vi "Helmholtz2D_Solve Lin Sys_Apply Corner.vi"(6 "Boundary Condition":cluster{"type":T2, "Value":dbl[]}[](array[cluster]) {"type" items=["Dirichlet", "Neumann"]}, 7 "Domain":T3={"x"={"start x"=0.0, "end x"=1.0, "# of x-points"=11}, "y"={"start y"=0.0, "end y"=1.0, "# of y-points"=11}}, 10 "D":T1, 11 "C'":T1) -> (0 "D' End Y":T1, 1 "D' Start Y":T1, 2 "C' End Y":T1, 3 "C' Start Y":T1)   [LabVIEW 2017, in "NI_PDE.lvlib"]
uses:
  <vilib>/gmath/NI_PDE.lvlib
  <vilib>/Analysis/Matrix/Datatypes/RealMatrix.ctl
  <vilib>/gmath/pde.llb/Common/PDE_BC Type.ctl
  <vilib>/Analysis/7linalg.llb/Create Special Real Matrix.vi
  <vilib>/Analysis/NI_AALPro.lvlib
  <vilib>/Analysis/Matrix/NI_Matrix.lvlib
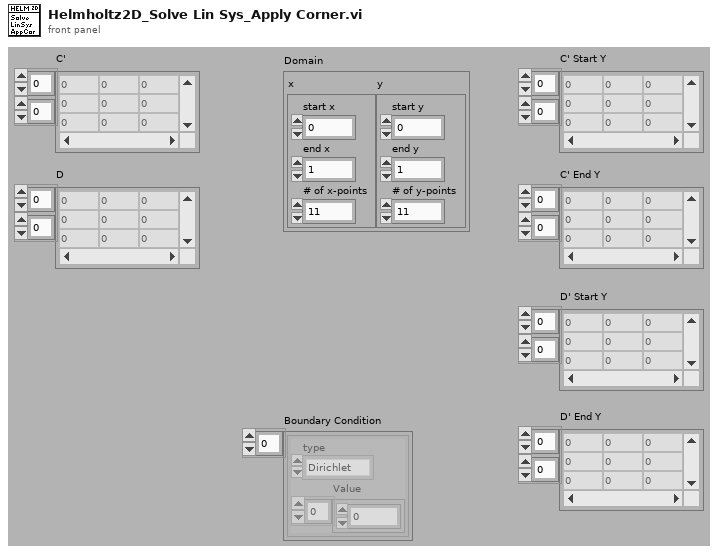
[diagram p1: front panel]
types:
  T1 = typedef "NI_Matrix.lvlib/RealMatrix.ctl" = dbl[][]
  T2 = typedef "NI_PDE.lvlib/PDE_BC Type.ctl" = i32
  T3 = cluster{"x":cluster{"start x":dbl, "end x":dbl, "# of x-points":i32}, "y":cluster{"start y":dbl, "end y":dbl, "# of y-points":i32}}
  T4 = enum32{"Identity", "Diagonal", "Toepliz", "Vandermonde", "Companion"}
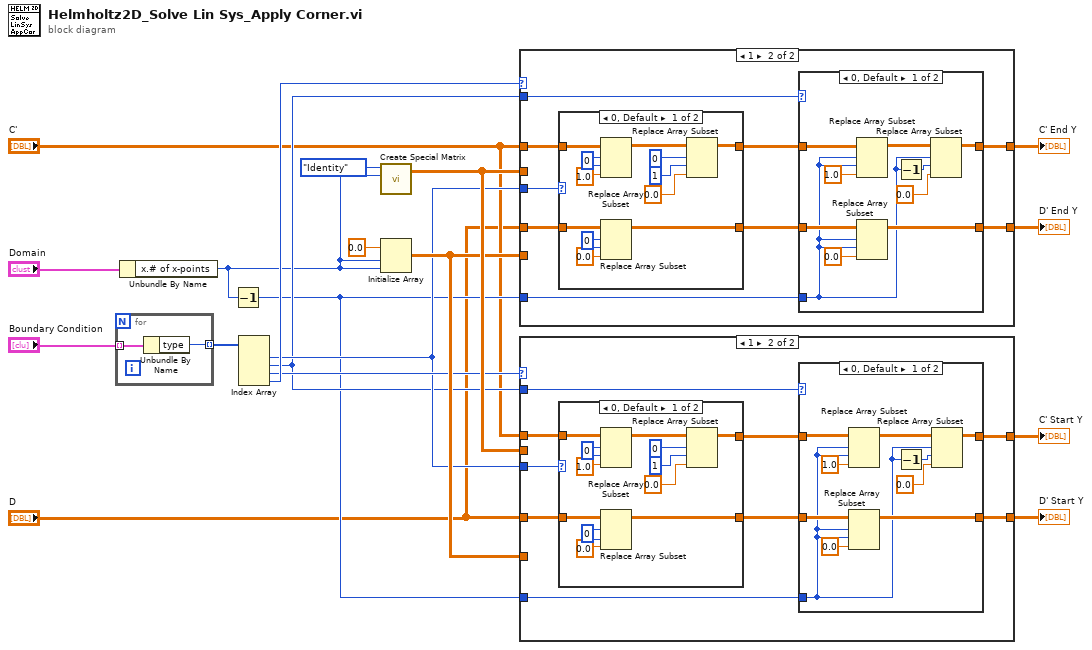
[diagram p0: block diagram]
diagram:
  n1 = for {
    tunnel: "Boundary Condition" -> [w21] mode=indexing
    tunnel: [w20] -> w9 mode=indexing
    n2 = Unbundle By Name(w21) -> ("type"=w20:T2)
  }
  n3 = Unbundle By Name("Domain") -> ("x.# of x-points"=w1:i32)
  n4 = Decrement(x=w1) -> (x-1=w4:i32)
  n5 = Index Array(array=w9) -> (element #1=w6:T2, element #2=w5:T2, element #3=w7:T2, element #4=w8:T2)  [unwired: 4 in]
  n6 = call-poly <vilib>:"Create Special Matrix.vi"("matrix type"=T4."Identity", "matrix size"=w1) -> ("Special Matrix"=w15:T1)  [unwired: 2 in, 2 out]
  n7 = Initialize Array(0.0 ("element"), w1, w1) -> (w14:dbl[][])
  n8 = case shown="1" w8 {
    tunnel: w15 -> [w23 _]
    tunnel: [w23 w27] -> w13
    tunnel: "C'" -> [_ w31]
    tunnel: w6 -> [_ w32]
    tunnel: "D" -> [_ w30]
    tunnel: [w22 w25] -> w12
    tunnel: w14 -> [w22 _]
    tunnel: w5 -> [_ w29]
    tunnel: w4 -> [_ w24]
    frame 0, Default {
    }
    frame 1 {
      n9 = case shown="0, Default" w32 {
        tunnel: w31 -> [w49 w58]
        tunnel: [w46 w58] -> w28
        tunnel: [w54 w57] -> w26
        tunnel: w30 -> [w55 w57]
        frame 0, Default {
          w48 = 0 ("index (row)")
          w45 = 0 ("index (row)")
          n10 = Replace Array Subset(array=w49, new element=1.0 ("new element/subarray"), index (row)=w48, index (col)=w48) -> (w47:T1)
          n11 = Replace Array Subset(array=w55, new element=0.0 ("new element/subarray"), index (row)=w45, index (col)=w45) -> (w54:T1)
          n12 = Replace Array Subset(array=w47, new element=0.0 ("new element/subarray"), index (row)=0, index (col)=1 ("index (row)")) -> (w46:T1)
        }
        frame 1 {
        }
      }
      n13 = case shown="0, Default" w29 {
        tunnel: w28 -> [w37 w44]
        tunnel: [w35 w44] -> w27
        tunnel: [w40 w43] -> w25
        tunnel: w26 -> [w41 w43]
        tunnel: w24 -> [w33 _]
        frame 0, Default {
          n14 = Replace Array Subset(array=w37, new element=1.0 ("new element/subarray"), index (row)=w33, index (col)=w33) -> (w36:T1)
          n15 = Replace Array Subset(array=w41, new element=0.0 ("new element/subarray"), index (row)=w33, index (col)=w33) -> (w40:T1)
          n16 = Decrement(x=w33) -> (x-1=w34:i32)
          n17 = Replace Array Subset(array=w36, new element=0.0 ("new element/subarray"), index (row)=w33, index (col)=w34) -> (w35:T1)
        }
        frame 1 {
        }
      }
    }
  }
  "D' End Y" <- w12
  "C' End Y" <- w13
  n18 = case shown="1" w7 {
    tunnel: w15 -> [w60 _]
    tunnel: [w60 w64] -> w11
    tunnel: "C'" -> [_ w68]
    tunnel: w6 -> [_ w69]
    tunnel: "D" -> [_ w67]
    tunnel: [w59 w62] -> w10
    tunnel: w14 -> [w59 _]
    tunnel: w5 -> [_ w66]
    tunnel: w4 -> [_ w61]
    frame 0, Default {
    }
    frame 1 {
      n19 = case shown="0, Default" w69 {
        tunnel: w68 -> [w86 w95]
        tunnel: [w83 w95] -> w65
        tunnel: [w91 w94] -> w63
        tunnel: w67 -> [w92 w94]
        frame 0, Default {
          w85 = 0 ("index (row)")
          w82 = 0 ("index (row)")
          n20 = Replace Array Subset(array=w86, new element=1.0 ("new element/subarray"), index (row)=w85, index (col)=w85) -> (w84:T1)
          n21 = Replace Array Subset(array=w92, new element=0.0 ("new element/subarray"), index (row)=w82, index (col)=w82) -> (w91:T1)
          n22 = Replace Array Subset(array=w84, new element=0.0 ("new element/subarray"), index (row)=0, index (col)=1 ("index (row)")) -> (w83:T1)
        }
        frame 1 {
        }
      }
      n23 = case shown="0, Default" w66 {
        tunnel: w65 -> [w74 w81]
        tunnel: [w72 w81] -> w64
        tunnel: [w77 w80] -> w62
        tunnel: w63 -> [w78 w80]
        tunnel: w61 -> [w70 _]
        frame 0, Default {
          n24 = Replace Array Subset(array=w74, new element=1.0 ("new element/subarray"), index (row)=w70, index (col)=w70) -> (w73:T1)
          n25 = Replace Array Subset(array=w78, new element=0.0 ("new element/subarray"), index (row)=w70, index (col)=w70) -> (w77:T1)
          n26 = Decrement(x=w70) -> (x-1=w71:i32)
          n27 = Replace Array Subset(array=w73, new element=0.0 ("new element/subarray"), index (row)=w70, index (col)=w71) -> (w72:T1)
        }
        frame 1 {
        }
      }
    }
  }
  "C' Start Y" <- w11
  "D' Start Y" <- w10
